vi "temperatureSetpointRequestView.vi"(10 "UserEvents in":refnum<class "UserEvents.lvclass">) -> ()   [LabVIEW 2013, in "AITDTViews.lvlib"]
uses:
  AITDTViews.lvlib
  UserEvents/UserEvents.lvclass
  CommandFactory/CommandFactory.lvclass
  UserEvents/UserEvents.lvclass/UserEvents.ctl
  Typedefs/StateSelector.ctl
  Typedefs/CommandSelector.ctl
  Typedefs/AITDTTypedefs.lvlib
panel:
  out "Temperature Setpoint To Apply":dbl[unit]=275.15 caption="Please set demand temperature to" min=271.15 max=275.15 format="%.1f"
  in  "setpointApplied":bool
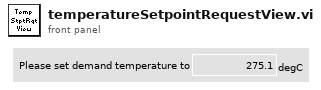
[diagram p1: front panel]
types:
  T1 = typedef "AITDTTypedefs.lvlib/PubDataEvents.ctl" = cluster{"State":refnum<user-event>, "ErrorCode":refnum<user-event>, "OutputData":refnum<user-event>, "InputData":refnum<user-event>, "TestStatus":refnum<user-event>, "LogPath":refnum<user-event>, "TemperatureSetpointRequest":refnum<user-event>, "TemperatureSettling":refnum<user-event>, "WaitTimeStatus":refnum<user-event>}
  T2 = typedef "AITDTTypedefs.lvlib/SubDataEvents.ctl" = cluster{"Command":refnum<user-event>}
  T3 = cluster{"Event Registration Refnum":refnum<event-registration>, "Event Registration Refnum":refnum<event-registration>}
  T4 = typedef "AITDTTypedefs.lvlib/StateSelector.ctl" = enum16{"AwaitingSetpointAcknowledgmentState", "EndingCycleState", "FaultState", "OffState", "PausingState", "RequestingNewSetpointState", "SamplingState", "SettlingState", "SoakingState", "StabilizingState", "StandbyState", "StoppedState", "TransitioningTemperatureState"}
  T5 = typedef "AITDTTypedefs.lvlib/CommandSelector.ctl" = enum16{"ClearError", "ConfirmSetpointApplied", "Exit", "StandBy", "Start", "StartTest", "StopTest", "Update"}
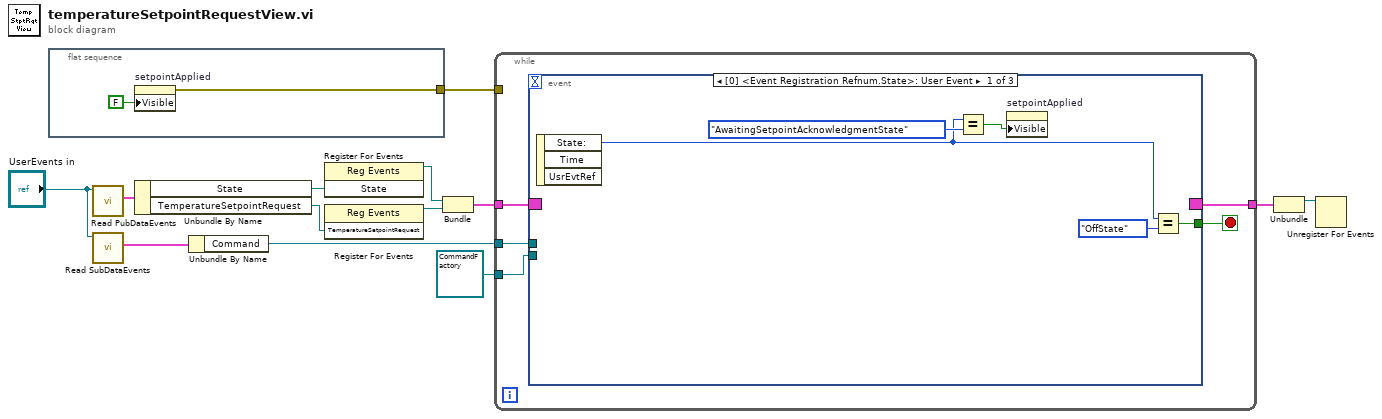
[diagram p0: block diagram]
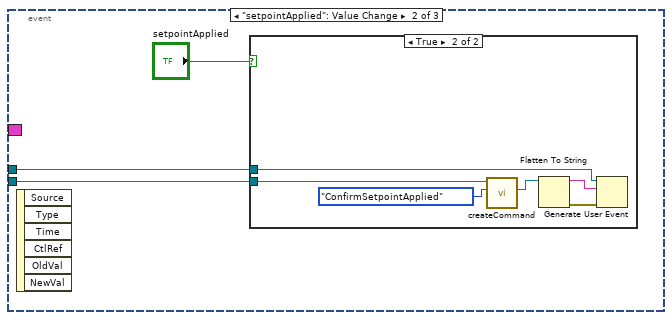
[diagram p2: hidden frame]
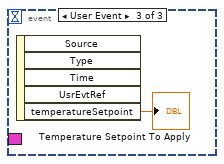
[diagram p4: hidden frame]
diagram:
  n1 = flat-sequence {
    tunnel: [w14] -> w3
    frame #0 {
      n2 = property on="setpointApplied" class="Bool"("Visible"=FALSE) -> (error out=w14:errorcluster)  [unwired: 2 in, 1 out]
    }
  }
  n3 = call "Read PubDataEvents.vi"("UserEvents in"="UserEvents in") -> ("PubDataEvents"=w10:T1)  [unwired: 9 in, 1 out]
  n4 = call "Read SubDataEvents.vi"("UserEvents in"="UserEvents in") -> ("SubDataEvents"=w11:T2)  [unwired: 9 in, 1 out]
  n5 = Unbundle By Name(w10) -> ("State"=w12:refnum<user-event>, "TemperatureSetpointRequest"=w2:refnum<user-event>)
  n6 = Unbundle By Name(w11) -> ("Command"=w8:refnum<user-event>)
  n7 = register-events(w12) -> (reference out=w13:refnum<event-registration>)  [unwired: 2 in, 1 out]
  n8 = register-events(w2) -> (reference out=w1:refnum<event-registration>)  [unwired: 2 in, 1 out]
  n9 = Bundle("Event Registration Refnum"=w13, "Event Registration Refnum"=w1) -> (w9:T3)  [unwired: 1 in]
  n10 = while {
    tunnel: w9 -> [w20]
    tunnel: w8 -> [w19]
    tunnel: [w18] -> w7
    tunnel: refnum<class "CommandFactory.lvclass"> refnum ("CommandFactory.lvclass") -> [w16]
    tunnel: w3 -> [_]
    stop <- w17 stop-if-true
    n11 = event shown="[0] <Event Registration Refnum.State>: User Event" {
      selector: w20 -> [_ _ _]
      dyn-events: [_ _ _] -> w18
      timeout: _ -> [_ _ _]
      tunnel: w19 -> [_ w27 _]
      tunnel: [w23 _ _] -> w17
      tunnel: w16 -> [_ w28 _]
      event User Event {
        n12 = event-data() -> ("State:"=w22:T4)  [unwired: 1 in, 2 out]
        n13 = Equal?(x=w22, y=StateSelector."AwaitingSetpointAcknowledgmentState") -> (x = y?=w21:bool)
        n14 = property on="setpointApplied" class="Bool"("Visible"=w21) -> ()  [unwired: 2 in, 2 out]
        n15 = Equal?(x=w22, y=StateSelector."OffState") -> (x = y?=w23:bool)
      }
      event "setpointApplied": Value Change {
        n16 = event-data() -> ()  [unwired: 1 in, 6 out]
        n17 = case shown="True" "setpointApplied" {
          tunnel: w28 -> [_ w34]
          tunnel: w27 -> [_ w33]
          frame False {
          }
          frame True {
            n18 = call-dynamic "createCommand.vi"("Command"=CommandSelector."ConfirmSetpointApplied", "CommandFactory in"=w34) -> ("command"=w29:refnum<class "Command.lvclass">)  [unwired: 7 in, 2 out]
            n19 = Flatten To String(anything=w29) -> (data string=w30:string, error out=w31:errorcluster)  [unwired: 3 in, 1 out]
            n20 = Generate User Event(user event=w33, event data cluster=w30, error in=w31) -> ()  [unwired: 1 in, 2 out]
          }
        }
      }
      event User Event {
        n21 = event-data() -> ("temperatureSetpoint"=→"Temperature Setpoint To Apply":dbl[unit])  [unwired: 1 in, 4 out]
      }
    }
  }
  n22 = Unbundle(w7) -> ("Event Registration Refnum"=w6:refnum<event-registration>)  [unwired: 1 out]
  n23 = Unregister For Events(event registration refnum=w6) -> ()  [unwired: 1 in, 1 out]
